vi "Process.vi"(11 "Initial Config":T1={"Log Files Directory"=path "", "Max Lines Per File"=10000}) -> ()   [LabVIEW 2020, in "Logger Actor.lvclass"]
uses:
  Logger Actor.lvclass
  Config.ctl
  Base Actor/Actor/Actor.lvclass/Actor.ctl
  Base Actor/Sequencer/Sequencer.lvclass/Sequencer.ctl
  Logger Actor.lvclass/Logger Actor.ctl
  <vilib>/Utility/High Resolution Relative Seconds.vi
  C:/dev/PGS/2001 - TBCM/Source/RT/RTAF/Source/RTAF/Actors/Base Actor/Actor/Actor.lvclass
  Base Actor/Actor/Actor.lvclass
  Log/Log.lvclass
panel:
  out "Iteration":i32
  in  "Tick Period [ms]":i32=5 min=2 step=1
  out "Tick Period [s]":dbl format="%.1p"
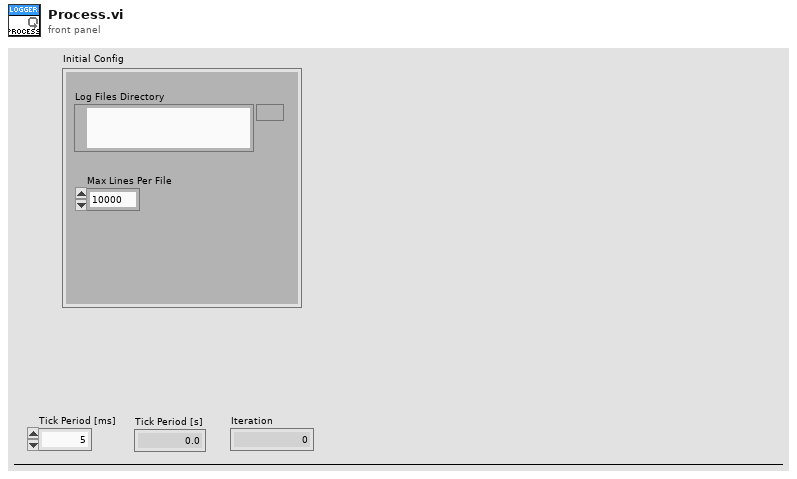
[diagram p1: front panel]
types:
  T1 = typedef "Logger Actor.lvclass/Config.ctl" = cluster{"Log Files Directory":path, "Max Lines Per File":i32}
  T2 = enum32{"Invalid", "Standard", "Closed", "Hidden", "Minimized", "Maximized"}
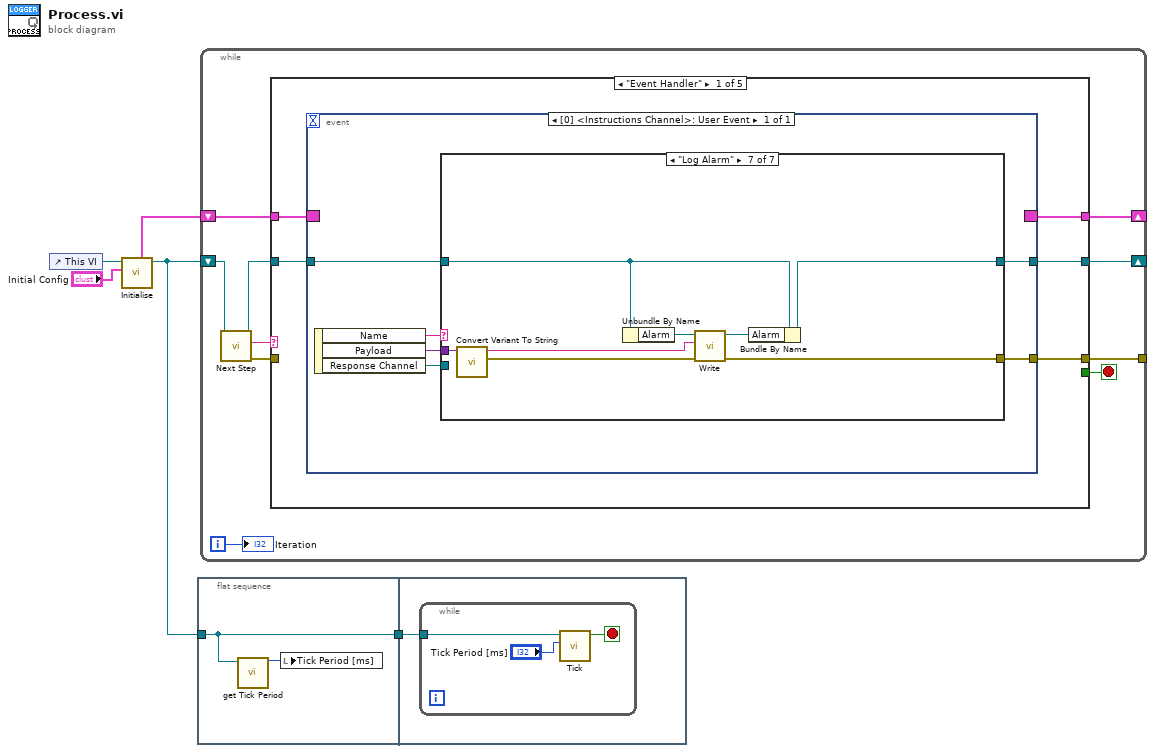
[diagram p0: block diagram]
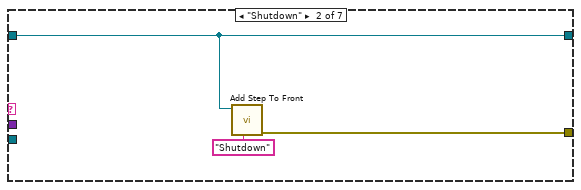
[diagram p3: hidden frame]
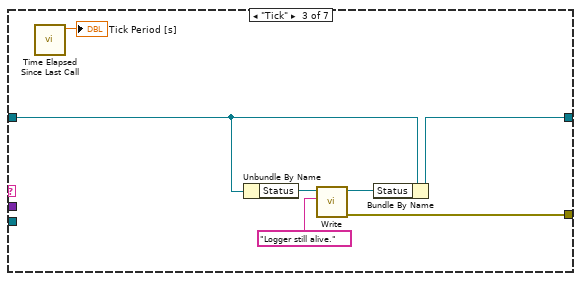
[diagram p4: hidden frame]
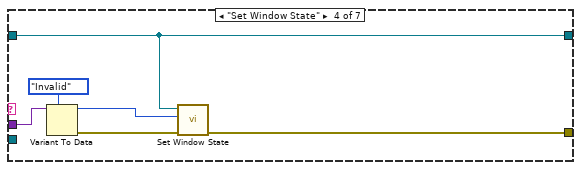
[diagram p5: hidden frame]
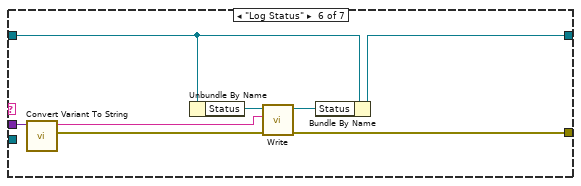
[diagram p7: hidden frame]
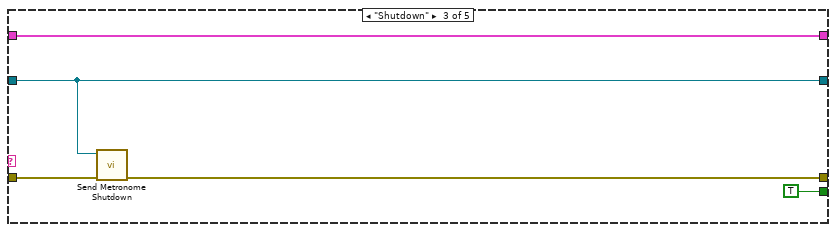
[diagram p9: hidden frame]
diagram:
  n1 = control-ref of="This VI"() -> (w2:refnum<vi>)
  n2 = call "Initialise.vi"("Initial Config"="Initial Config", "Process"=w2) -> ("Actor out"=w5:refnum<class "Logger Actor.lvclass">, "Mailboxes"=w3:cluster{"Mailbox":refnum<event-registration>})  [unwired: 7 in, 1 out]
  n3 = flat-sequence {
    tunnel: w5 -> [w7]
    tunnel: [w7] -> w4
    tunnel: w4 -> [w8]
    frame #0 {
      n4 = call "get Tick Period.vi"("Actor in"=w7) -> ("Tick Period [ms]"=w6:i32)  [unwired: 10 in]
      n5 = local write "Tick Period [ms]"(w6) -> ()
    }
    frame #1 {
      n6 = while {
        tunnel: w8 -> [w11]
        stop <- w9 stop-if-true
        n7 = call "Tick.vi"("Tick Period [ms]"="Tick Period [ms]", "Actor in"=w11) -> ("Shutdown"=w9:bool)  [unwired: 9 in]
      }
    }
  }
  n8 = while {
    shift-right: [w20] -> _
    shift-left: w5 -> [w17]
    tunnel: [w19] -> _
    shift-right: [w12] -> _
    shift-left: w3 -> [w21]
    i -> [w13]
    stop <- w14 stop-if-true
    n9 = call "Next Step.vi"("Actor in"=w17) -> ("error out"=w18:errorcluster, "Next Step"=w15:string, "Actor out"=w16:refnum<class "Logger Actor.lvclass">)  [unwired: 8 in]
    n10 = case shown="\"Event Handler\"" w15 {
      tunnel: w21 -> [w26 w67 w70 w75 w78]
      tunnel: [_ _ TRUE _ _] -> w14
      tunnel: w16 -> [w25 w69 w73 w77 w80]
      tunnel: [w24 w69 w73 w77 w80] -> w20
      tunnel: [w23 w68 w72 w76 w79] -> w19
      tunnel: w18 -> [_ w68 w71 w76 w79]
      tunnel: [w22 w67 w70 w75 w78] -> w12
      frame "Event Handler" {
        n11 = event shown="[0] <Instructions Channel>: User Event" {
          selector: w26 -> [_]
          dyn-events: [_] -> w22
          timeout: _ -> [_]
          tunnel: w25 -> [w30]
          tunnel: [w29] -> w24
          tunnel: [w27] -> w23
          event User Event {
            n12 = event-data() -> ("Name"=w32:string, "Payload"=w31:variant, "Response Channel"=w28:refnum<notifier>)  [unwired: 1 in]
            n13 = case shown="\"Log Alarm\"" w32 {
              tunnel: w31 -> [_ _ _ w49 _ w53 w61]
              tunnel: w30 -> [w33 w36 w39 w46 w50 w55 w63]
              tunnel: [w33 w36 w40 w46 w50 w56 w64] -> w29
              tunnel: w28 -> [_ _ _ _ _ _ _]
              tunnel: [_ w35 w41 w47 _ w58 w66] -> w27
              frame Default {
              }
              frame "Shutdown" {
                n14 = call "Add Step To Front.vi"("Step Name"="Shutdown", "Actor in"=w36) -> ("error out"=w35:errorcluster)  [unwired: 9 in]
              }
              frame "Tick" {
                n15 = call "Time Elapsed Since Last Call.vi"() -> ("Time Elapsed Since Last Call [s]"=→"Tick Period [s]":dbl)  [unwired: 11 in]
                n16 = Unbundle By Name(w39) -> ("Status"=w42:refnum<class "Log.lvclass">)
                n17 = call "Write.vi"("Message"="Logger still alive.", "Log in"=w42) -> ("error out"=w41:errorcluster, "Log out"=w43:refnum<class "Log.lvclass">)  [unwired: 8 in]
                n18 = Bundle By Name(cluster=w39, "Status"=w43) -> (w40:refnum<class "Logger Actor.lvclass">)
              }
              frame "Set Window State" {
                n19 = Variant To Data(type=T2."Invalid", Variant=w49) -> (data=w45:T2, error out=w48:errorcluster)  [unwired: 1 in]
                n20 = call "Set Window State.vi"("error in (no error)"=w48, "State"=w45, "Actor in"=w46) -> ("error out"=w47:errorcluster)  [unwired: 8 in]
              }
              frame "----------------------------------" {
              }
              frame "Log Status" {
                n21 = call "Convert Variant To String.vi"("Variant"=w53) -> ("error out"=w51:errorcluster, "String"=w52:string)  [unwired: 9 in]
                n22 = Unbundle By Name(w55) -> ("Status"=w54:refnum<class "Log.lvclass">)
                n23 = call "Write.vi"("error in (no error)"=w51, "Message"=w52, "Log in"=w54) -> ("error out"=w58:errorcluster, "Log out"=w57:refnum<class "Log.lvclass">)  [unwired: 7 in]
                n24 = Bundle By Name(cluster=w55, "Status"=w57) -> (w56:refnum<class "Logger Actor.lvclass">)
              }
              frame "Log Alarm" {
                n25 = call "Convert Variant To String.vi"("Variant"=w61) -> ("error out"=w59:errorcluster, "String"=w60:string)  [unwired: 9 in]
                n26 = Unbundle By Name(w63) -> ("Alarm"=w62:refnum<class "Log.lvclass">)
                n27 = call "Write.vi"("error in (no error)"=w59, "Message"=w60, "Log in"=w62) -> ("error out"=w66:errorcluster, "Log out"=w65:refnum<class "Log.lvclass">)  [unwired: 7 in]
                n28 = Bundle By Name(cluster=w63, "Alarm"=w65) -> (w64:refnum<class "Logger Actor.lvclass">)
              }
            }
          }
        }
      }
      frame "Error Handler" {
      }
      frame "Shutdown" {
        n29 = call "Send Metronome Shutdown.vi"("error in (no error)"=w71, "Actor in"=w73) -> ("error out"=w72:errorcluster)  [unwired: 9 in]
      }
      frame "Unhandled Step", Default {
      }
      frame "-----------------------------------" {
      }
    }
    "Iteration" <- w13
  }
